vi "matrici_v44.vi"() -> ()   [LabVIEW 2009]
uses:
  <vilib>/Native 3D Graph/xcontrol/3DPC_SurfacePlot.xctl
  <vilib>/Native 3D Graph/classes/Line/Line.lvclass
panel:
  in  "Domeniul de definitie y":dbl(slide)=0.5242070116861437 scale=-2.0..2.0
  out "3D Graph":refnum<class "Base Datatype.lvclass">[](xcontrol)
  out "X":dbl=3.390233722871455
  out "y":dbl=-3.1847650123943945
  in  "stop":bool
  in  "Domeniul de definitie x":dbl(slide)=6.780467445742905 scale=-10.0..10.0
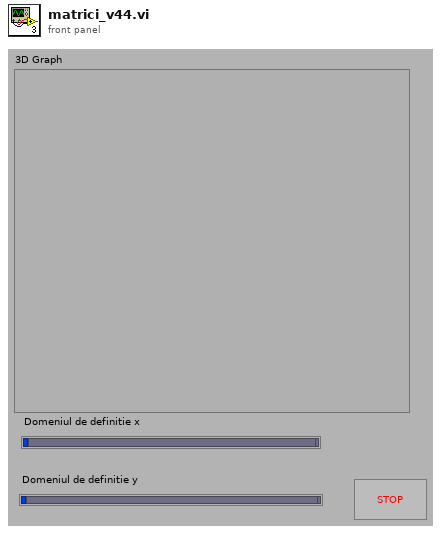
[diagram p1: front panel]
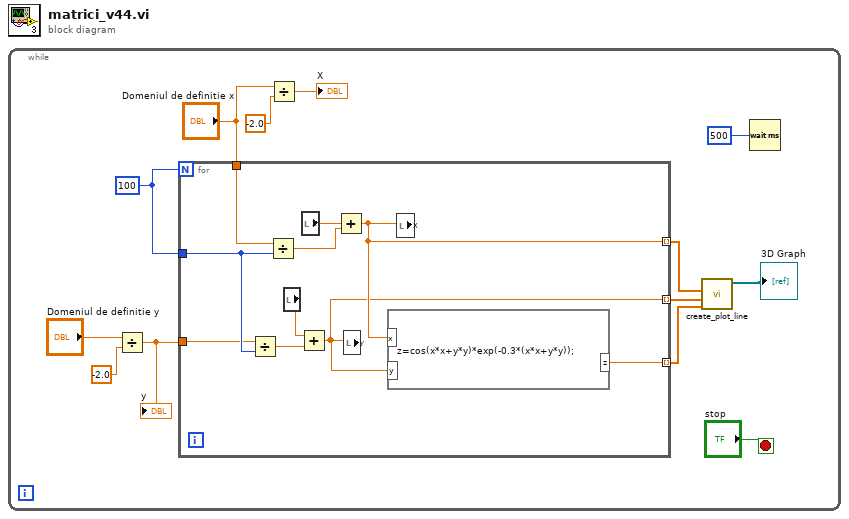
[diagram p0: block diagram]
diagram:
  n1 = while {
    stop <- "stop" stop-if-true
    w11 = 100
    n2 = Divide(x="Domeniul de definitie y", y=-2.0) -> (x/y=w1:dbl)
    "y" <- w1
    n3 = for {
      N: w11 -> [_]
      tunnel: [w19] -> w9 mode=indexing
      tunnel: w11 -> [w16]
      tunnel: "Domeniul de definitie x" -> [w22]
      tunnel: [w18] -> w8 mode=indexing
      tunnel: [w17] -> w7 mode=indexing
      tunnel: w1 -> [w14]
      n4 = Divide(x=w14, y=w16) -> (x/y=w15:dbl)
      n5 = Divide(x=w22, y=w16) -> (x/y=w20:dbl)
      n6 = local read "y"() -> (w21:dbl)
      n7 = Add(x=w21, y=w15) -> (x+y=w17:dbl)
      n8 = local read "X"() -> (w23:dbl)
      n9 = Add(x=w23, y=w20) -> (x+y=w19:dbl)
      n10 = local write "y"(w17) -> ()
      n11 = formula code="z=cos(x*x+y*y)*exp(-0.3*(x*x+y*y));"("x"=w19, "y"=w17) -> ("z"=w18:dbl)
      n12 = local write "X"(w19) -> ()
    }
    n13 = Divide(x="Domeniul de definitie x", y=-2.0) -> (x/y=→"X":dbl)
    n14 = call <vilib>:"create_plot_line.vi"("z vector"=w8, "y vector"=w7, "x vector"=w9) -> ("plots out"=→"3D Graph":refnum<class "Base Datatype.lvclass">[])  [unwired: 2 in, 6 out]
    n15 = Wait (ms)(milliseconds to wait=500) -> ()  [unwired: 1 out]
  }
